vi "setUp.vi"(8 "error in (no error)":errorcluster, 11 "reference in":refnum<class "Instrument Addon Error System Tests.lvclass">) -> (0 "error out":errorcluster, 3 "reference out":refnum<class "Instrument Addon Error System Tests.lvclass">)   [LabVIEW 2018, in "Instrument Addon Error System Tests.lvclass"]
doc: "setUp runs prior to the test method during test execution. Use this method to initialize any object data required by your tests."
uses:
  Instrument Addon Error System Tests.lvclass
  C:/Program Files (x86)/National Instruments/LabVIEW 2018/vi.lib/addons/_JKI Toolkits/VI Tester/TestCase.llb/TestCase.lvclass
  <vilib>/addons/_JKI Toolkits/VI Tester/TestCase.llb/TestCase.lvclass
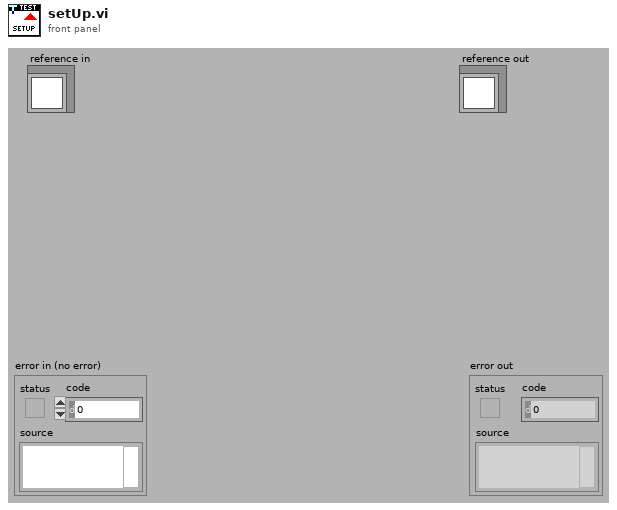
[diagram p1: front panel]
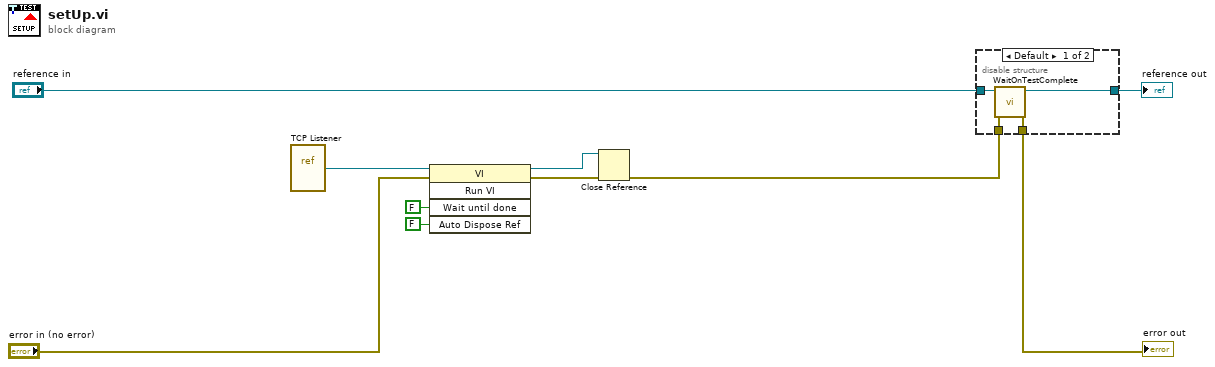
[diagram p0: block diagram]
diagram:
  n1 = vi-ref "TCP Listener.vi"() -> (w7:refnum<vi>)
  n2 = invoke class="VI" method="Run VI"(reference=w7, error in="error in (no error)", "Wait until done"=FALSE ("Wait Until Done"), "Auto Dispose Ref"=FALSE ("Auto Dispose Reference")) -> (reference out=w6:refnum<vi>, error out=w5:errorcluster)  [unwired: 1 in, 3 out]
  n3 = Close Reference(reference=w6, error in (no error)=w5) -> (error out=w4:errorcluster)
  n4 = disable-structure shown="Default" {
    disable-tunnel: w4 -> [w14 w15]
    disable-tunnel: [w13 w15] -> w10
    disable-tunnel: [w12 w16] -> w9
    disable-tunnel: "reference in" -> [w11 w16]
    frame condition #0 (active) {
      n5 = call <vilib>:"WaitOnTestComplete.vi"("error in (no error)"=w14, "TestCase in"=w11) -> ("error out"=w13:errorcluster, "TestCase out"=w12:refnum<class "Instrument Addon Error System Tests.lvclass">)  [unwired: 8 in]
    }
    frame condition #1 {
    }
  }
  "error out" <- w10
  "reference out" <- w9
